vi "DataLog Values of Prior Points.vi"(1 "times":dbl[](array[numeric]) format="%<%H:%M:%S%2u\n%Y/%m/%d>T", 2 "points":T1[](array[typedef]) {"value" format="%.3e"; "time" format="%<%H:%M:%S%2u\n%Y/%m/%d>T"}) -> (0 "prior values":dbl[](array[numeric]))   [LabVIEW 2012]
doc: "Serves the interpolation of set&hold tags. Given an array of times (which need not be ordered) find the values of prior points (last point with timestamp <= the specified time). The timestamps of the points are assumed to increase monotonically. Times that lie before the time range of the points result in a NaN value. Times that lie after the time range of the points result in the value of the last point. The algorithm scales as O(T*log(P)) where T is the number of times and P the number of points."
uses:
  typedefs/clusters/t_DataLog Point.ctl
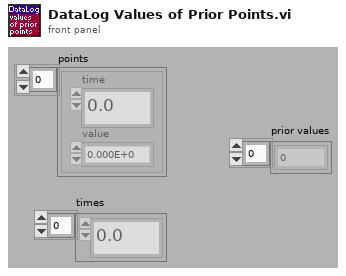
[diagram p1: front panel]
types:
  T1 = typedef "t_DataLog Point.ctl" = cluster{"time":dbl, "value":dbl}
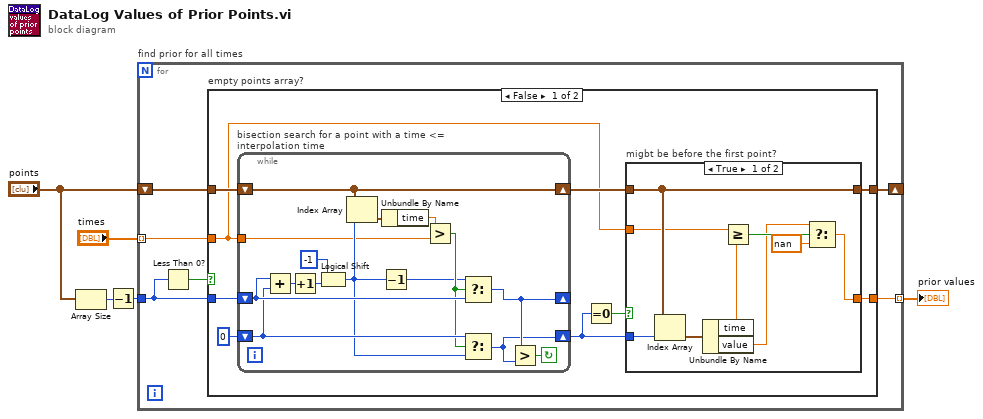
[diagram p0: block diagram]
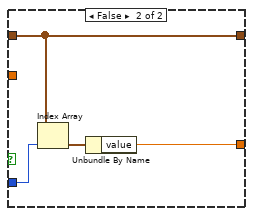
[diagram p2: hidden frame]
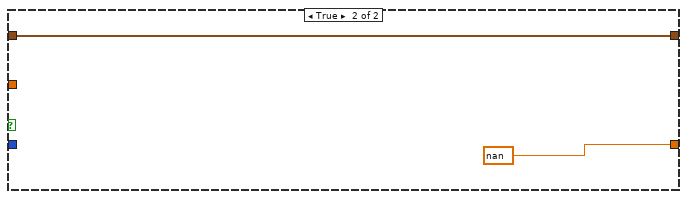
[diagram p3: hidden frame]
diagram:
  n1 = Array Size(array="points") -> (size(s)=w5:i32)
  n2 = Decrement(x=w5) -> (x-1=w4:i32)
  n3 = for "find prior for all times" {
    tunnel: w4 -> [w7]
    tunnel: "times" -> [w10] mode=indexing
    shift-right: [w9] -> _
    shift-left: "points" -> [w11]
    tunnel: [w6] -> w1 mode=indexing
    n4 = Less Than 0?(x=w7) -> (x < 0?=w8:bool)
    n5 = case "empty points array?" shown="False" w8 {
      tunnel: w7 -> [w19 _]
      tunnel: w11 -> [w18 w49]
      tunnel: w10 -> [w13 _]
      tunnel: [w14 w49] -> w9
      tunnel: [w16 nan ("value")] -> w6
      frame False {
        n6 = while "bisection search for a point with a time <= interpolation time" {
          shift-right: [w40] -> w12
          shift-left: 0 -> [w47]
          shift-right: [w46] -> _
          shift-left: w19 -> [w48]
          tunnel: w13 -> [w37]
          shift-right: [w34] -> w17
          shift-left: w18 -> [w34]
          stop <- w45 continue-if-true
          n7 = Add(x=w48, y=w47) -> (x+y=w43:i32)
          n8 = Increment(x=w43) -> (x+1=w38:i32)
          n9 = Logical Shift(y=-1, x=w38) -> (x << y=w41:i32)
          n10 = Index Array(array=w34, index=w41) -> (element=w36:T1)
          n11 = Decrement(x=w41) -> (x-1=w39:i32)
          n12 = Unbundle By Name(w36) -> ("time"=w35:dbl)
          n13 = Greater?(x=w35, y=w37) -> (0:w44:bool)
          n14 = Select(t=w39, s=w44, f=w48) -> (s? t:f=w46:i32)
          n15 = Select(t=w47, s=w44, f=w41) -> (s? t:f=w40:i32)
          n16 = Greater?(x=w46, y=w40) -> (0:w45:bool)
        }
        n17 = Equal To 0?(x=w12) -> (x = 0?=w15:bool)
        n18 = case "migbt be before the first point?" shown="True" w15 {
          tunnel: w17 -> [w27 w30]
          tunnel: w12 -> [w28 w32]
          tunnel: [w21 w31] -> w16
          tunnel: [w27 w30] -> w14
          tunnel: w13 -> [w26 _]
          frame True {
            n19 = Index Array(array=w27, index=w28) -> (element=w29:T1)
            n20 = Unbundle By Name(w29) -> ("time"=w25:dbl, "value"=w23:dbl)
            n21 = Greater Or Equal?(x=w26, y=w25) -> (x >= y?=w24:bool)
            n22 = Select(t=w23, s=w24, f=nan) -> (s? t:f=w21:dbl)
          }
          frame False {
            n23 = Index Array(array=w30, index=w32) -> (element=w33:T1)
            n24 = Unbundle By Name(w33) -> ("value"=w31:dbl)
          }
        }
      }
      frame True {
      }
    }
  }
  "prior values" <- w1
